vi "tone_info.vi"(8 "error in (no error)":errorcluster, 9 "Center Freq":dbl=0.1, 10 "threshold":dbl=0.1, 11 "time signal in":waveform(dbl)) -> (0 "error out":errorcluster, 2 "amplitude":dbl, 3 "frequency":dbl)   [LabVIEW 2011]
uses:
  <vilib>/measure/matone.llb/Extract Multiple Tone Information 1 Chan.vi
  <vilib>/measure/NI_MAPro.lvlib
panel:
  out "element":T1
  out "multiple tone information":T2(array[cluster]) {"detected phase (deg)" format="%_6g"; "detected amplitude" format="%_6p"; "detected frequency" format="%_6p"}
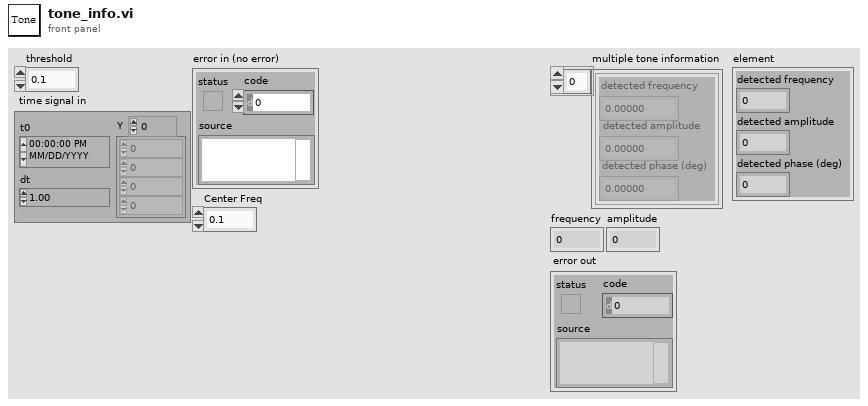
[diagram p1: front panel]
types:
  T1 = cluster{"detected frequency":dbl, "detected amplitude":dbl, "detected phase (deg)":dbl}
  T2 = cluster{"detected frequency":dbl, "detected amplitude":dbl, "detected phase (deg)":dbl}[]
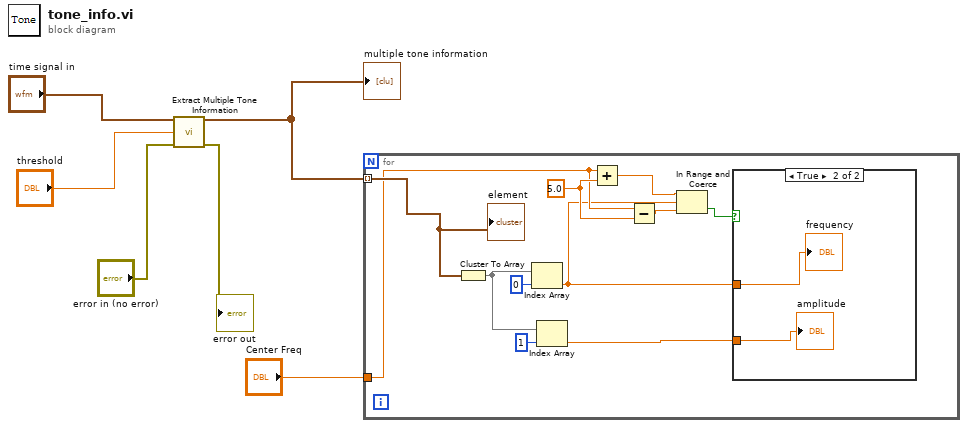
[diagram p0: block diagram]
diagram:
  n1 = call-poly <vilib>:"Extract Multiple Tone Information.vi"("time signal in"="time signal in", "threshold"="threshold", "error in (no error)"="error in (no error)") -> ("multiple tone information"=w5:T2, "error out"=→"error out":errorcluster)  [unwired: 10 in, 1 out]
  "multiple tone information" <- w5
  n2 = for {
    tunnel: w5 -> [w14] mode=indexing
    tunnel: "Center Freq" -> [w10]
    w11 = 5.0 ("y")
    n3 = Cluster To Array(cluster=w14) -> (array=w17:dbl[])
    n4 = Index Array(array=w17, index=0) -> (element=w7:dbl)
    n5 = Index Array(array=w17, index=1) -> (element=w8:dbl)
    n6 = Add(x=w10, y=w11) -> (x+y=w13:dbl)
    n7 = Subtract(x=w10, y=w11) -> (x-y=w12:dbl)
    n8 = In Range and Coerce(upper limit=w13, x=w7, lower limit=w12) -> (In Range?=w9:bool)  [unwired: 1 out]
    n9 = case shown="True" w9 {
      tunnel: w8 -> [_ w19]
      tunnel: w7 -> [_ w18]
      frame False {
      }
      frame True {
        "amplitude" <- w19
        "frequency" <- w18
      }
    }
    "element" <- w14
  }
